vi "_script_fix_Parse State Queue in Find Parse State Queue vi name.vi"   [LabVIEW 2014]
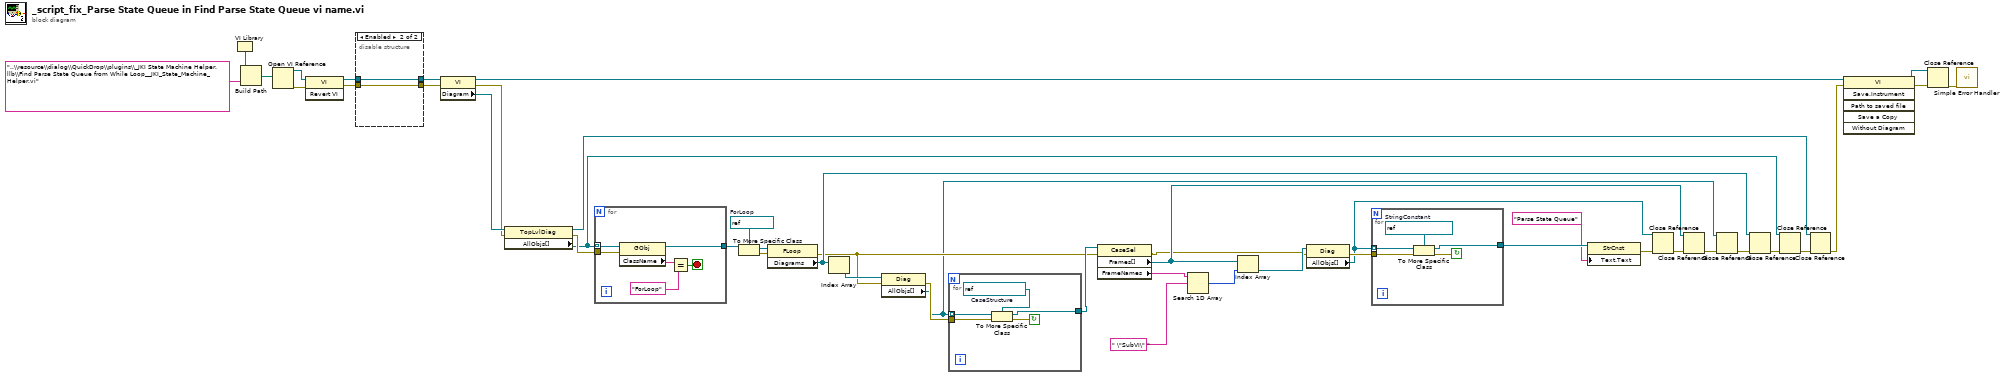
[diagram p0: block diagram]
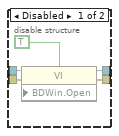
[diagram p2: hidden frame]
diagram:
  w32 = refnum<vi> refnum  # ForLoop
  n1 = VI Library() -> (path=w43:path)
  n2 = Build Path(base path=w43, name or relative path="..\\resource\\dialog\\QuickDrop\\plugins\\_JKI State Machine Helper.llb\\Find Parse State Queue from While Loop__JKI_State_Machine_Helper.vi") -> (appended path=w41:path)
  n3 = Open VI Reference(vi path=w41) -> (vi reference=w44:refnum<vi>, error out=w45:errorcluster)  [unwired: 5 in]
  n4 = invoke class="VI" method="Revert VI"(reference=w44, error in=w45) -> (reference out=w19:refnum<vi>, error out=w18:errorcluster)  [unwired: 1 in, 1 out]
  n5 = disable-structure shown="Enabled" {
    disable-tunnel: w19 -> [w50 w52]
    disable-tunnel: w18 -> [w49 w51]
    disable-tunnel: [w48 w52] -> w17
    disable-tunnel: [w47 w51] -> w16
    frame Disabled {
      n6 = property class="VI"(reference=w50, error in=w49, "BDWin.Open"=TRUE ("Block Diagram Window:Open")) -> (reference out=w48:refnum<vi>, error out=w47:errorcluster)
    }
    frame Enabled {
    }
  }
  n7 = property class="VI"(reference=w17, error in=w16) -> (reference out=w40:refnum<vi>, error out=w35:errorcluster, "Diagram"=w36:refnum<vi>)
  n8 = property class="TopLvlDiag"(reference=w36, error in=w35) -> (reference out=w21:refnum<vi>, error out=w34:errorcluster, "AllObjs[]"=w23:refnum<vi>[])
  n9 = for {
    tunnel: w23 -> [w58] mode=indexing
    tunnel: w34 -> [w57]
    tunnel: [w56] -> w33
    stop <- w53 stop-if-true
    n10 = property class="GObj"(reference=w58, error in=w57) -> (reference out=w56:refnum<vi>, "ClassName"=w55:string)  [unwired: 1 out]
    n11 = Equal?(x=w55, y="ForLoop") -> (x = y?=w53:bool)
  }
  n12 = To More Specific Class(target class=w32, reference=w33) -> (specific class reference=w31:refnum<vi>, error out=w30:errorcluster)  [unwired: 1 in]
  n13 = property class="FLoop"(reference=w31, error in=w30) -> (error out=w11:errorcluster, "Diagrams"=w15:refnum<vi>[])  [unwired: 1 out]
  n14 = Index Array(array=w15) -> (element=w14:refnum<vi>)  [unwired: 1 in]
  n15 = property class="Diag"(reference=w14, error in=w11) -> (error out=w13:errorcluster, "AllObjs[]"=w7:refnum<vi>[])  [unwired: 1 out]
  n16 = for {
    tunnel: w7 -> [w63] mode=indexing
    tunnel: w13 -> [w62]
    tunnel: [w60] -> w12
    stop <- w61 continue-if-true
    w59 = refnum<vi> refnum  # CaseStructure
    n17 = To More Specific Class(target class=w59, reference=w63, error in=w62) -> (specific class reference=w60:refnum<vi>, error out=w61:errorcluster)
  }
  n18 = property class="CaseSel"(reference=w12, error in=w11) -> (error out=w1:errorcluster, "Frames[]"=w4:refnum<vi>[], "FrameNames"=w6:string[])  [unwired: 1 out]
  n19 = Search 1D Array(1D array=w6, element=" \"SubVI\" " ("y")) -> (index of element=w3:i32)  [unwired: 1 in]
  n20 = Index Array(array=w4, index=w3) -> (element=w2:refnum<vi>)
  n21 = property class="Diag"(reference=w2, error in=w1) -> (error out=w29:errorcluster, "AllObjs[]"=w25:refnum<vi>[])  [unwired: 1 out]
  n22 = for {
    tunnel: w25 -> [w68] mode=indexing
    tunnel: w29 -> [w67]
    tunnel: [w64] -> w28
    stop <- w65 continue-if-true
    w66 = refnum<vi> refnum  # StringConstant
    n23 = To More Specific Class(target class=w66, reference=w68, error in=w67) -> (specific class reference=w64:refnum<vi>, error out=w65:errorcluster)
  }
  n24 = property class="StrCnst"(reference=w28, "Text.Text"="Parse State Queue") -> (error out=w26:errorcluster)  [unwired: 1 in, 1 out]
  n25 = Close Reference(reference=w25, error in (no error)=w26) -> (error out=w10:errorcluster)
  n26 = Close Reference(reference=w4, error in (no error)=w10) -> (error out=w9:errorcluster)
  n27 = Close Reference(reference=w7, error in (no error)=w9) -> (error out=w8:errorcluster)
  n28 = Close Reference(reference=w15, error in (no error)=w8) -> (error out=w24:errorcluster)
  n29 = Close Reference(reference=w23, error in (no error)=w24) -> (error out=w22:errorcluster)
  n30 = Close Reference(reference=w21, error in (no error)=w22) -> (error out=w20:errorcluster)
  n31 = invoke class="VI" method="Save.Instrument"(reference=w40, error in=w20) -> (reference out=w38:refnum<vi>, error out=w39:errorcluster)  [unwired: 4 in, 4 out]
  n32 = Close Reference(reference=w38, error in (no error)=w39) -> (error out=w37:errorcluster)
  n33 = call <vilib>:"Simple Error Handler.vi"("error in (no error)"=w37) -> ()  [unwired: 4 in, 5 out]
